vi "HFRR ADV v010new software.vi"() -> ()   [LabVIEW 2025] (continued)
              n1799 = String Subset(string=w2117, offset (0)=45, length (rest)=9 ("length (rest)")) -> (substring=w2132:string)
              n1800 = String Subset(string=w2117, offset (0)=65, length (rest)=9 ("length (rest)")) -> (substring=w2138:string)
              n1801 = Fract/Exp String To Number(string=w2124) -> (number=w2121:dbl)  [unwired: 3 in, 1 out]
              n1802 = Fract/Exp String To Number(string=w2118) -> (number=w2116:dbl)  [unwired: 3 in, 1 out]
              n1803 = Fract/Exp String To Number(string=w2126) -> (number=w2125:dbl)  [unwired: 3 in, 1 out]
              n1804 = Fract/Exp String To Number(string=w2132) -> (number=w2129:dbl)  [unwired: 3 in, 1 out]
              n1805 = Fract/Exp String To Number(string=w2138) -> (number=w2135:dbl)  [unwired: 3 in, 1 out]
              n1806 = Add(x=w2135, y=0.0) -> (x+y=w2133:dbl)
            }
            n1807 = for {
              N: w1987 -> [_]
              tunnel: w1998 -> [w2078]
              tunnel: w1997 -> [w2077]
              tunnel: [w2067] -> w1956 mode=indexing
              tunnel: [w2065] -> w1954 mode=indexing
              tunnel: [w2066] -> w1950 mode=indexing
              tunnel: w1985 -> [_]
              tunnel: [w2059] -> w1952 mode=indexing
              tunnel: [w2055] -> w1934 mode=indexing
              tunnel: [w2051] -> w1910 mode=indexing
              tunnel: [w2048] -> w1891 mode=indexing
              tunnel: [w2044] -> w1850 mode=indexing
              (unwired) 9 ("length (rest)")
              (unwired) 9 ("length (rest)")
              (unwired) TRUE ("line mode (F)")
              n1808 = Read from Text File "Read File"(file (use dialog)=w2077, error in=w2078) -> (text=w2045:string)  [unwired: 2 in, 3 out]
              n1809 = local write "String 8"(w2045) -> ()
              n1810 = String Subset(string=w2045, offset (0)=85) -> (substring=w2047:string)  [unwired: 1 in]
              n1811 = String Subset(string=w2045, offset (0)=35, length (rest)=9 ("length (rest)")) -> (substring=w2068:string)
              n1812 = String Subset(string=w2045, offset (0)=55, length (rest)=9 ("length (rest)")) -> (substring=w2053:string)
              n1813 = String Subset(string=w2045, offset (0)=25) -> (substring=w2049:string)  [unwired: 1 in]
              n1814 = String Subset(string=w2045, offset (0)=15, length (rest)=9 ("length (rest)")) -> (substring=w2074:string)
              n1815 = String Subset(string=w2045, offset (0)=0, length (rest)=14 ("length (rest)")) -> (substring=w2071:string)
              n1816 = String Subset(string=w2045, offset (0)=45, length (rest)=9 ("length (rest)")) -> (substring=w2058:string)
              n1817 = String Subset(string=w2045, offset (0)=65, length (rest)=9 ("length (rest)")) -> (substring=w2064:string)
              n1818 = Fract/Exp String To Number(string=w2047) -> (number=w2044:dbl)  [unwired: 3 in, 1 out]
              n1819 = Fract/Exp String To Number(string=w2068) -> (number=w2066:dbl)  [unwired: 3 in, 1 out]
              n1820 = Fract/Exp String To Number(string=w2053) -> (number=w2051:dbl)  [unwired: 3 in, 1 out]
              n1821 = Fract/Exp String To Number(string=w2049) -> (number=w2048:dbl)  [unwired: 3 in, 1 out]
              n1822 = Fract/Exp String To Number(string=w2074) -> (number=w2065:dbl)  [unwired: 3 in, 1 out]
              n1823 = Fract/Exp String To Number(string=w2071) -> (number=w2067:dbl)  [unwired: 3 in, 1 out]
              n1824 = Fract/Exp String To Number(string=w2058) -> (number=w2055:dbl)  [unwired: 3 in, 1 out]
              n1825 = Fract/Exp String To Number(string=w2064) -> (number=w2061:dbl)  [unwired: 3 in, 1 out]
              n1826 = Add(x=w2061, y=0.0) -> (x+y=w2059:dbl)
            }
            n1827 = String To Path(string=w1904) -> (path=w2002:path)
            n1828 = String To Path(string=w1902) -> (path=w1996:path)
            n1829 = local read "Numeric 11"() -> (w1986:i32)
            n1830 = local read "Numeric 13"() -> (w1988:i32)
            n1831 = Open/Create/Replace File "Open File"(file path (use dialog)=w2002) -> (refnum out=w2000:refnum<file>, error out=w1999:errorcluster)  [unwired: 5 in, 1 out]
            n1832 = Open/Create/Replace File "Open File"(file path (use dialog)=w1996) -> (refnum out=w1995:refnum<file>, error out=w1994:errorcluster)  [unwired: 5 in, 1 out]
            n1833 = for {
              N: w1986 -> [_]
              tunnel: w2000 -> [w2115]
              tunnel: w1999 -> [w2114]
              tunnel: [w2104] -> w1966 mode=indexing
              tunnel: [w2102] -> w1964 mode=indexing
              tunnel: [w2103] -> w1959 mode=indexing
              tunnel: w1985 -> [_]
              tunnel: [w2096] -> w1961 mode=indexing
              tunnel: [w2092] -> w1937 mode=indexing
              tunnel: [w2088] -> w1912 mode=indexing
              tunnel: [w2084] -> w1893 mode=indexing
              tunnel: [w2079] -> w1851 mode=indexing
              (unwired) TRUE ("line mode (F)")
              n1834 = Read from Text File "Read File"(file (use dialog)=w2115, error in=w2114) -> (text=w2080:string)  [unwired: 2 in, 3 out]
              n1835 = local write "String 7"(w2080) -> ()
              n1836 = String Subset(string=w2080, offset (0)=85, length (rest)=9 ("length (rest)")) -> (substring=w2083:string)
              n1837 = String Subset(string=w2080, offset (0)=35, length (rest)=9 ("length (rest)")) -> (substring=w2105:string)
              n1838 = String Subset(string=w2080, offset (0)=55, length (rest)=9 ("length (rest)")) -> (substring=w2091:string)
              n1839 = String Subset(string=w2080, offset (0)=25, length (rest)=9 ("length (rest)")) -> (substring=w2085:string)
              n1840 = String Subset(string=w2080, offset (0)=45, length (rest)=9 ("length (rest)")) -> (substring=w2093:string)
              n1841 = String Subset(string=w2080, offset (0)=0, length (rest)=14 ("length (rest)")) -> (substring=w2108:string)
              n1842 = String Subset(string=w2080, offset (0)=15, length (rest)=9 ("length (rest)")) -> (substring=w2111:string)
              n1843 = String Subset(string=w2080, offset (0)=65, length (rest)=9 ("length (rest)")) -> (substring=w2097:string)
              n1844 = Fract/Exp String To Number(string=w2083) -> (number=w2079:dbl)  [unwired: 3 in, 1 out]
              n1845 = Fract/Exp String To Number(string=w2105) -> (number=w2103:dbl)  [unwired: 3 in, 1 out]
              n1846 = Fract/Exp String To Number(string=w2091) -> (number=w2088:dbl)  [unwired: 3 in, 1 out]
              n1847 = Fract/Exp String To Number(string=w2085) -> (number=w2084:dbl)  [unwired: 3 in, 1 out]
              n1848 = Fract/Exp String To Number(string=w2093) -> (number=w2092:dbl)  [unwired: 3 in, 1 out]
              n1849 = Fract/Exp String To Number(string=w2108) -> (number=w2104:dbl)  [unwired: 3 in, 1 out]
              n1850 = Fract/Exp String To Number(string=w2111) -> (number=w2102:dbl)  [unwired: 3 in, 1 out]
              n1851 = Fract/Exp String To Number(string=w2097) -> (number=w2100:dbl)  [unwired: 3 in, 1 out]
              n1852 = Add(x=w2100, y=0.0) -> (x+y=w2096:dbl)
            }
            n1853 = for {
              N: w1988 -> [_]
              tunnel: w1995 -> [w2043]
              tunnel: w1994 -> [w2042]
              tunnel: [w2032] -> w1948 mode=indexing
              tunnel: [w2031] -> w1941 mode=indexing
              tunnel: w1985 -> [_]
              tunnel: [w2020] -> w1946 mode=indexing
              tunnel: [w2025] -> w1943 mode=indexing
              tunnel: [w2021] -> w1933 mode=indexing
              tunnel: [w2016] -> w1908 mode=indexing
              tunnel: [w2012] -> w1889 mode=indexing
              tunnel: [w2007] -> w1849 mode=indexing
              (unwired) 1.0 ("x")
              (unwired) TRUE ("line mode (F)")
              n1854 = Read from Text File "Read File"(file (use dialog)=w2043, error in=w2042) -> (text=w2008:string)  [unwired: 2 in, 3 out]
              n1855 = local write "String 12"(w2008) -> ()
              n1856 = String Subset(string=w2008, offset (0)=85, length (rest)=9 ("length (rest)")) -> (substring=w2010:string)
              n1857 = String Subset(string=w2008, offset (0)=35, length (rest)=9 ("length (rest)")) -> (substring=w2033:string)
              n1858 = String Subset(string=w2008, offset (0)=55, length (rest)=9 ("length (rest)")) -> (substring=w2018:string)
              n1859 = String Subset(string=w2008, offset (0)=25, length (rest)=9 ("length (rest)")) -> (substring=w2014:string)
              n1860 = String Subset(string=w2008, offset (0)=45, length (rest)=9 ("length (rest)")) -> (substring=w2023:string)
              n1861 = String Subset(string=w2008, offset (0)=15, length (rest)=9 ("length (rest)")) -> (substring=w2039:string)
              n1862 = String Subset(string=w2008, offset (0)=0, length (rest)=14 ("length (rest)")) -> (substring=w2036:string)
              n1863 = String Subset(string=w2008, offset (0)=65, length (rest)=9 ("length (rest)")) -> (substring=w2026:string)
              n1864 = Fract/Exp String To Number(string=w2010) -> (number=w2007:dbl)  [unwired: 3 in, 1 out]
              n1865 = Fract/Exp String To Number(string=w2033) -> (number=w2031:dbl)  [unwired: 3 in, 1 out]
              n1866 = Fract/Exp String To Number(string=w2018) -> (number=w2016:dbl)  [unwired: 3 in, 1 out]
              n1867 = Fract/Exp String To Number(string=w2014) -> (number=w2012:dbl)  [unwired: 3 in, 1 out]
              n1868 = Fract/Exp String To Number(string=w2023) -> (number=w2021:dbl)  [unwired: 3 in, 1 out]
              n1869 = Fract/Exp String To Number(string=w2039) -> (number=w2020:dbl)  [unwired: 3 in, 1 out]
              n1870 = Fract/Exp String To Number(string=w2036) -> (number=w2032:dbl)  [unwired: 3 in, 1 out]
              n1871 = Fract/Exp String To Number(string=w2026) -> (number=w2029:dbl)  [unwired: 3 in, 1 out]
              n1872 = Add(x=w2029, y=0.0) -> (x+y=w2025:dbl)
            }
            n1873 = Delete From Array(array=w1891, index=0) -> (array with subset deleted=w1864:dbl[])  [unwired: 1 in, 1 out]
            n1874 = Delete From Array(array=w1954, index=0) -> (array with subset deleted=w1927:dbl[])  [unwired: 1 in, 1 out]
            n1875 = Delete From Array(array=w1934, index=0) -> (array with subset deleted=w1922:dbl[])  [unwired: 1 in, 1 out]
            n1876 = Delete From Array(array=w1952, index=0) -> (array with subset deleted=w1953:dbl[])  [unwired: 1 in, 1 out]
            n1877 = call-poly <vilib>:"Mean.vi"("X"=w1864) -> ("mean"=→"КОФ2 4":dbl)  [unwired: 1 out]
            n1878 = call-poly <vilib>:"Mean.vi"("X"=w1927) -> ("mean"=→"КОФ3":dbl)  [unwired: 1 out]
            n1879 = call-poly <vilib>:"Mean.vi"("X"=w1922) -> ("mean"=→"CP3":dbl)  [unwired: 1 out]
            n1880 = Delete From Array(array=w1916, index=0) -> (array with subset deleted=w1843:dbl[])  [unwired: 1 in, 1 out]
            n1881 = Delete From Array(array=w1855, index=0) -> (array with subset deleted=w1842:dbl[])  [unwired: 1 in, 1 out]
            n1882 = Delete From Array(array=w1895, index=0) -> (array with subset deleted=w1866:dbl[])  [unwired: 1 in, 1 out]
            n1883 = Delete From Array(array=w1973, index=0) -> (array with subset deleted=w1928:dbl[])  [unwired: 1 in, 1 out]
            n1884 = Delete From Array(array=w1939, index=0) -> (array with subset deleted=w1924:dbl[])  [unwired: 1 in, 1 out]
            "array w/ subset deleted" <- w1924
            n1885 = Delete From Array(array=w1970, index=0) -> (array with subset deleted=w1971:dbl[])  [unwired: 1 in, 1 out]
            n1886 = call-poly <vilib>:"Mean.vi"("X"=w1866) -> ("mean"=→"КОФ2 2":dbl)  [unwired: 1 out]
            n1887 = call-poly <vilib>:"Mean.vi"("X"=w1928) -> ("mean"=→"КОФ1":dbl)  [unwired: 1 out]
            n1888 = Bundle "Bundle"(w1843, w1842) -> (w1848:cluster{dbl[], dbl[]})  [unwired: 1 in]
            n1889 = Bundle "Bundle"(w1843, w1971) -> (w1835:cluster{dbl[], dbl[]})  [unwired: 1 in]
            n1890 = Delete From Array(array=w1850, index=0) -> (array with subset deleted=w1838:dbl[])  [unwired: 1 in, 1 out]
            n1891 = Delete From Array(array=w1851, index=0) -> (array with subset deleted=w1840:dbl[])  [unwired: 1 in, 1 out]
            n1892 = Delete From Array(array=w1961, index=0) -> (array with subset deleted=w1962:dbl[])  [unwired: 1 in, 1 out]
            n1893 = Delete From Array(array=w1849, index=0) -> (array with subset deleted=w1836:dbl[])  [unwired: 1 in, 1 out]
            n1894 = Delete From Array(array=w1943, index=0) -> (array with subset deleted=w1944:dbl[])  [unwired: 1 in, 1 out]
            n1895 = Delete From Array(array=w1968, index=0) -> (array with subset deleted=w1874:dbl[])  [unwired: 1 in, 1 out]
            n1896 = Delete From Array(array=w1914, index=0) -> (array with subset deleted=w1870:dbl[])  [unwired: 1 in, 1 out]
            n1897 = Delete From Array(array=w1950, index=0) -> (array with subset deleted=w1872:dbl[])  [unwired: 1 in, 1 out]
            n1898 = Delete From Array(array=w1910, index=0) -> (array with subset deleted=w1868:dbl[])  [unwired: 1 in, 1 out]
            n1899 = Delete From Array(array=w1959, index=0) -> (array with subset deleted=w1873:dbl[])  [unwired: 1 in, 1 out]
            n1900 = Delete From Array(array=w1912, index=0) -> (array with subset deleted=w1869:dbl[])  [unwired: 1 in, 1 out]
            n1901 = Delete From Array(array=w1893, index=0) -> (array with subset deleted=w1865:dbl[])  [unwired: 1 in, 1 out]
            n1902 = Delete From Array(array=w1937, index=0) -> (array with subset deleted=w1923:dbl[])  [unwired: 1 in, 1 out]
            n1903 = Delete From Array(array=w1964, index=0) -> (array with subset deleted=w1925:dbl[])  [unwired: 1 in, 1 out]
            n1904 = Delete From Array(array=w1941, index=0) -> (array with subset deleted=w1871:dbl[])  [unwired: 1 in, 1 out]
            n1905 = Delete From Array(array=w1908, index=0) -> (array with subset deleted=w1867:dbl[])  [unwired: 1 in, 1 out]
            n1906 = Delete From Array(array=w1889, index=0) -> (array with subset deleted=w1863:dbl[])  [unwired: 1 in, 1 out]
            n1907 = Delete From Array(array=w1933, index=0) -> (array with subset deleted=w1921:dbl[])  [unwired: 1 in, 1 out]
            n1908 = Delete From Array(array=w1946, index=0) -> (array with subset deleted=w1926:dbl[])  [unwired: 1 in, 1 out]
            n1909 = Delete From Array(array=w1956, index=0) -> (array with subset deleted=w1839:dbl[])  [unwired: 1 in, 1 out]
            n1910 = Delete From Array(array=w1966, index=0) -> (array with subset deleted=w1841:dbl[])  [unwired: 1 in, 1 out]
            n1911 = Delete From Array(array=w1948, index=0) -> (array with subset deleted=w1837:dbl[])  [unwired: 1 in, 1 out]
            n1912 = Bundle "Bundle"(w1843, w1874) -> (w1861:cluster{dbl[], dbl[]})  [unwired: 1 in]
            n1913 = Bundle "Bundle"(w1843, w1928) -> (w1862:cluster{dbl[], dbl[]})  [unwired: 1 in]
            n1914 = Bundle "Bundle"(w1874, w1870) -> (w1876:cluster{dbl[], dbl[]})  [unwired: 1 in]
            n1915 = Bundle "Bundle"(w1839, w1838) -> (w1846:cluster{dbl[], dbl[]})  [unwired: 1 in]
            n1916 = Bundle "Bundle"(w1872, w1868) -> (w1878:cluster{dbl[], dbl[]})  [unwired: 1 in]
            n1917 = Bundle "Bundle"(w1839, w1872) -> (w1982:cluster{dbl[], dbl[]})  [unwired: 1 in]
            n1918 = Bundle "Bundle"(w1839, w1868) -> (w1906:cluster{dbl[], dbl[]})  [unwired: 1 in]
            n1919 = Bundle "Bundle"(w1839, w1927) -> (w1992:cluster{dbl[], dbl[]})  [unwired: 1 in]
            n1920 = Bundle "Bundle"(w1839, w1922) -> (w1930:cluster{dbl[], dbl[]})  [unwired: 1 in]
            n1921 = Bundle "Bundle"(w1839, w1953) -> (w1977:cluster{dbl[], dbl[]})  [unwired: 1 in]
            n1922 = Bundle "Bundle"(w1873, w1869) -> (w1877:cluster{dbl[], dbl[]})  [unwired: 1 in]
            n1923 = Bundle "Bundle"(w1841, w1840) -> (w1847:cluster{dbl[], dbl[]})  [unwired: 1 in]
            n1924 = Bundle "Bundle"(w1841, w1873) -> (w1984:cluster{dbl[], dbl[]})  [unwired: 1 in]
            n1925 = Bundle "Bundle"(w1841, w1869) -> (w1907:cluster{dbl[], dbl[]})  [unwired: 1 in]
            n1926 = Bundle "Bundle"(w1841, w1923) -> (w1931:cluster{dbl[], dbl[]})  [unwired: 1 in]
            n1927 = Bundle "Bundle"(w1841, w1925) -> (w1993:cluster{dbl[], dbl[]})  [unwired: 1 in]
            n1928 = Bundle "Bundle"(w1841, w1962) -> (w1975:cluster{dbl[], dbl[]})  [unwired: 1 in]
            n1929 = Bundle "Bundle"(w1871, w1867) -> (w1879:cluster{dbl[], dbl[]})  [unwired: 1 in]
            n1930 = Bundle "Bundle"(w1837, w1836) -> (w1845:cluster{dbl[], dbl[]})  [unwired: 1 in]
            n1931 = Bundle "Bundle"(w1837, w1871) -> (w1983:cluster{dbl[], dbl[]})  [unwired: 1 in]
            n1932 = Bundle "Bundle"(w1837, w1867) -> (w1905:cluster{dbl[], dbl[]})  [unwired: 1 in]
            n1933 = Bundle "Bundle"(w1837, w1921) -> (w1929:cluster{dbl[], dbl[]})  [unwired: 1 in]
            n1934 = Bundle "Bundle"(w1837, w1926) -> (w1991:cluster{dbl[], dbl[]})  [unwired: 1 in]
            n1935 = Bundle "Bundle"(w1837, w1944) -> (w1976:cluster{dbl[], dbl[]})  [unwired: 1 in]
            n1936 = call-poly <vilib>:"Mean.vi"("X"=w1924) -> ("mean"=→"CP1":dbl)  [unwired: 1 out]
            n1937 = call-poly <vilib>:"Mean.vi"("X"=w1865) -> ("mean"=→"КОФ2 3":dbl)  [unwired: 1 out]
            n1938 = call-poly <vilib>:"Mean.vi"("X"=w1923) -> ("mean"=→"CP2":dbl)  [unwired: 1 out]
            n1939 = call-poly <vilib>:"Mean.vi"("X"=w1925) -> ("mean"=→"КОФ2":dbl)  [unwired: 1 out]
            n1940 = call-poly <vilib>:"Mean.vi"("X"=w1863) -> ("mean"=→"КОФ2 5":dbl)  [unwired: 1 out]
            n1941 = call-poly <vilib>:"Mean.vi"("X"=w1921) -> ("mean"=→"CP4":dbl)  [unwired: 1 out]
            n1942 = call-poly <vilib>:"Mean.vi"("X"=w1926) -> ("mean"=→"КОФ4":dbl)  [unwired: 1 out]
            n1943 = Bundle "Bundle"(w1843, w1870) -> (w1834:cluster{dbl[], dbl[]})  [unwired: 1 in]
            n1944 = Bundle "Bundle"(w1843, w1924) -> (w1857:cluster{dbl[], dbl[]})  [unwired: 1 in]
            n1945 = Build Array "Build Array"(w1834, w1857) -> (w1860:cluster{dbl[], dbl[]}[])
            "XY Graph 17" <- w1860
            n1946 = Build Array "Build Array"(w1848, w1847, w1846, w1845) -> (→"Frequency ( Hz )":cluster{dbl[], dbl[]}[])
            n1947 = Build Array "Build Array"(w1876, w1877, w1878, w1879) -> (→"Air Temp ( °C ) vs Humidity ( % RH )":cluster{dbl[], dbl[]}[])
            n1948 = Build Array "Build Array"(w1861, w1984, w1982, w1983) -> (→"Air Temperature  ( °C )":cluster{dbl[], dbl[]}[])
            n1949 = Build Array "Build Array"(w1834, w1907, w1906, w1905) -> (→"Humidity ( %RH )":cluster{dbl[], dbl[]}[])
            n1950 = Build Array "Build Array"(w1862, w1993, w1992, w1991) -> (→"Coefficient Of Friction":cluster{dbl[], dbl[]}[])
            n1951 = Build Array "Build Array"(w1857, w1931, w1930, w1929) -> (→"Sample Temperature ( °C )":cluster{dbl[], dbl[]}[])
            n1952 = Build Array "Build Array"(w1835, w1975, w1977, w1976) -> (→"XY Graph 13":cluster{dbl[], dbl[]}[])
            n1953 = Bundle "Bundle"(w1843, w1866) -> (w1888:cluster{dbl[], dbl[]})  [unwired: 1 in]
            n1954 = Bundle "Bundle"(w1839, w1864) -> (w1886:cluster{dbl[], dbl[]})  [unwired: 1 in]
            n1955 = Bundle "Bundle"(w1841, w1865) -> (w1887:cluster{dbl[], dbl[]})  [unwired: 1 in]
            n1956 = Bundle "Bundle"(w1837, w1863) -> (w1885:cluster{dbl[], dbl[]})  [unwired: 1 in]
            n1957 = Build Array "Build Array"(w1888, w1887, w1886, w1885) -> (→"Stroke ( mm )":cluster{dbl[], dbl[]}[])
            n1958 = local write "XY Graph 16"(w1860) -> ()
          }
          frame #2 {
          }
          frame #3 {
            n1959 = local write "Numeric 8"(0 ("Numeric 8")) -> ()
            n1960 = local write "Numeric 11"(0 ("Numeric 11")) -> ()
            n1961 = local write "Numeric 12"(0 ("Numeric 12")) -> ()
            n1962 = local write "Numeric 13"(0 ("Numeric 13")) -> ()
            n1963 = property on="OPEN" class="Bool (strict)"("Visible"=TRUE) -> ()  [unwired: 2 in, 2 out]
            n1964 = local read "String Control 2"() -> (w2160:string)
            n1965 = local read "String Control 4"() -> (w2159:string)
            n1966 = local read "String Control 6"() -> (w2158:string)
            n1967 = local read "String Control 8"() -> (w2157:string)
            n1968 = Match Pattern(string=w2160, regular expression="Samples / cycle :- ") -> (after substring=w2174:string)  [unwired: 1 in, 3 out]
            n1969 = Match Pattern(string=w2160, regular expression="Frequency :- ") -> (after substring=w2193:string)  [unwired: 1 in, 3 out]
            n1970 = Match Pattern(string=w2159, regular expression="Samples / cycle :- ") -> (after substring=w2170:string)  [unwired: 1 in, 3 out]
            n1971 = Match Pattern(string=w2159, regular expression="Frequency :- ") -> (after substring=w2188:string)  [unwired: 1 in, 3 out]
            n1972 = Match Pattern(string=w2158, regular expression="Samples / cycle :- ") -> (after substring=w2166:string)  [unwired: 1 in, 3 out]
            n1973 = Match Pattern(string=w2158, regular expression="Frequency :- ") -> (after substring=w2183:string)  [unwired: 1 in, 3 out]
            n1974 = Match Pattern(string=w2157, regular expression="Samples / cycle :- ") -> (after substring=w2162:string)  [unwired: 1 in, 3 out]
            n1975 = Match Pattern(string=w2157, regular expression="Frequency :- ") -> (after substring=w2178:string)  [unwired: 1 in, 3 out]
            n1976 = String Subset(string=w2174, length (rest)=6 ("length (rest)")) -> (substring=w2176:string)  [unwired: 1 in]
            n1977 = String Subset(string=w2193, length (rest)=9 ("length (rest)")) -> (substring=w2195:string)  [unwired: 1 in]
            n1978 = String Subset(string=w2170, length (rest)=6 ("length (rest)")) -> (substring=w2172:string)  [unwired: 1 in]
            n1979 = String Subset(string=w2188, length (rest)=9 ("length (rest)")) -> (substring=w2190:string)  [unwired: 1 in]
            n1980 = String Subset(string=w2166, length (rest)=6 ("length (rest)")) -> (substring=w2168:string)  [unwired: 1 in]
            n1981 = String Subset(string=w2183, length (rest)=9 ("length (rest)")) -> (substring=w2185:string)  [unwired: 1 in]
            n1982 = String Subset(string=w2162, length (rest)=6 ("length (rest)")) -> (substring=w2164:string)  [unwired: 1 in]
            n1983 = String Subset(string=w2178, length (rest)=9 ("length (rest)")) -> (substring=w2180:string)  [unwired: 1 in]
            n1984 = Fract/Exp String To Number(string=w2176) -> (number=w2156:dbl)  [unwired: 3 in, 1 out]
            n1985 = Fract/Exp String To Number(string=w2195) -> (number=w2196:dbl)  [unwired: 3 in, 1 out]
            n1986 = Fract/Exp String To Number(string=w2172) -> (number=w2155:dbl)  [unwired: 3 in, 1 out]
            n1987 = Fract/Exp String To Number(string=w2190) -> (number=w2191:dbl)  [unwired: 3 in, 1 out]
            n1988 = Fract/Exp String To Number(string=w2168) -> (number=w2154:dbl)  [unwired: 3 in, 1 out]
            n1989 = Fract/Exp String To Number(string=w2185) -> (number=w2186:dbl)  [unwired: 3 in, 1 out]
            n1990 = Fract/Exp String To Number(string=w2164) -> (number=w2153:dbl)  [unwired: 3 in, 1 out]
            n1991 = Fract/Exp String To Number(string=w2180) -> (number=w2181:dbl)  [unwired: 3 in, 1 out]
            n1992 = local write "sample1"(w2156) -> ()
            n1993 = local write "freq1"(w2196) -> ()
            n1994 = local write "sample2"(w2155) -> ()
            n1995 = local write "freq2"(w2191) -> ()
            n1996 = local write "sample3"(w2154) -> ()
            n1997 = local write "freq3"(w2186) -> ()
            n1998 = local write "sample4"(w2153) -> ()
            n1999 = local write "freq 4"(w2181) -> ()
          }
        }
      }
    }
    n2000 = case shown="True" w1645 {
      selector: w1645 -> [_ w1773]
      frame False {
      }
      frame True {
        n2001 = Not(x=w1773) -> (.not. x?=w1769:bool)
        n2002 = local write "service 3"(w1769) -> ()
        n2003 = local write "OPEN 6"(w1769) -> ()
        n2004 = call <vilib>:"System Exec.vi"("wait until completion? (T)"=TRUE, "command line"="C:\\LAB-IQ\\Scar View.exe") -> ("error out"=→"error out 5":errorcluster)  [unwired: 6 in, 3 out]
      }
    }
    n2005 = case shown="\"Acquire\", Default" w1656 {
      frame "Acquire", Default {
        w2669 = 0.2 ("y")
        w2674 = 1.0 ("y")
        w2675 = 0.8 ("y")
        # "Elapsed time\ncof\nstroke\nAir temp\nTemp\nHumidity"
        n2006 = disable-structure shown="Disabled" {
          frame Disabled {
            n2007 = local read "Flag"() -> (w2692:dbl)
            n2008 = local read "RUN"() -> (w2689:bool)
            n2009 = Not(x=w2689) -> (.not. x?=w2688:bool)
            n2010 = Equal?(x=w2692, y=10.0) -> (x = y?=w2690:bool)
            n2011 = And(x=w2690, y=w2688) -> (x .and. y?=w2687:bool)
            n2012 = case shown="True" w2687 {
              frame False {
              }
              frame True {
                w2693 = FALSE ("Heater Button")
                n2013 = local write "Humidity"(w2693) -> ()
                n2014 = local write "Heater Button"(w2693) -> ()
              }
            }
          }
          frame Enabled {
          }
        }
        n2015 = disable-structure shown="Disabled" {
          frame Disabled {
            n2016 = case shown="True" {
              selector: _ -> [_ _]
              frame False {
              }
              frame True {
                w2784 = TRUE ("Heater")
                n2017 = local write "Humidity"(w2784) -> ()
                n2018 = local write "Heater Button"(w2784) -> ()
                n2019 = local read "TEST STANDARD"() -> (w2787:T3)
                n2020 = local read "TEST STANDARD"() -> (w2782:T3)
                n2021 = Equal?(x=w2787, y=enum16{"ASTM D6079", "ISO 12156", "Custom"}."ISO 12156" ("Test Standard")) -> (x = y?=w2785:bool)
                n2022 = Equal?(x=w2782, y=enum16{"ASTM D6079", "ISO 12156", "Custom"}."ASTM D6079" ("Test Standard")) -> (x = y?=w2781:bool)
                n2023 = case shown="True" w2785 {
                  frame False {
                  }
                  frame True {
                    n2024 = local write "Heater"(TRUE ("Heater")) -> ()
                    n2025 = local write "airtempflg"(FALSE ("airtempflg")) -> ()
                  }
                }
                n2026 = case shown="True" w2781 {
                  frame False {
                  }
                  frame True {
                    n2027 = local write "Heater"(FALSE ("Heater")) -> ()
                    n2028 = local write "airtempflg"(TRUE ("airtempflg")) -> ()
                  }
                }
              }
            }
          }
          frame Enabled {
          }
        }
        n2029 = stacked-sequence {
          frame #0 {
            n2030 = case shown="True" "RST FF" {
              frame False {
              }
              frame True {
                w2850 = 0.0 ("X Scale.Range:Maximum")
                n2031 = property on="Frictional Force ( N )" class="WFChart (strict)"("XScale.Maximum"=600.0 ("X Scale.Range:Maximum"), "XScale.Minimum"=w2850, "YScale.Maximum"=10.0 ("Y Scale.Range:Maximum"), "YScale.Minimum"=w2850) -> ()  [unwired: 2 in, 2 out]
              }
            }
          }
          frame #1 {
            n2032 = case shown="True" "RST TEMP" {
              frame False {
              }
              frame True {
                n2033 = property on="Temperature ( Deg C )" class="WFChart (strict)"("XScale.Minimum"=0.0 ("X Scale.Range:Minimum"), "XScale.Maximum"=600.0 ("X Scale.Range:Maximum"), "YScale.Minimum"=0.0 ("Y Scale.Range:Minimum"), "YScale.Maximum"=100.0 ("Y Scale.Range:Maximum")) -> ()  [unwired: 2 in, 2 out]
              }
            }
          }
          frame #2 {
            n2034 = case shown="True" "RSTCOF" {
              frame False {
              }
              frame True {
                n2035 = property on="Coefficient of Friction" class="WFChart (strict)"("XScale.Minimum"=0.0 ("X Scale.Range:Minimum"), "XScale.Maximum"=600.0 ("X Scale.Range:Maximum"), "YScale.Maximum"=1.0 ("X Scale.Range:Minimum"), "YScale.Minimum"=0.0 ("X Scale.Range:Minimum")) -> ()  [unwired: 2 in, 2 out]
              }
            }
          }
          frame #3 {
            n2036 = case shown="True" "RSTCOF 2" {
              frame False {
              }
              frame True {
                (unwired) 100.0 ("Y Scale.Range:Maximum")
                (unwired) 0.0 ("Y Scale.Range:Minimum")
                (unwired) 600.0 ("X Scale.Range:Maximum")
                (unwired) 0.0 ("X Scale.Range:Minimum")
              }
            }
          }
          frame #4 {
            n2037 = case shown="True" "RSTCOF 3" {
              frame False {
              }
              frame True {
                n2038 = property on="Electrical Contact Resistance ( % )" class="WFChart (strict)"("XScale.Minimum"=0.0 ("X Scale.Range:Minimum"), "XScale.Maximum"=600.0 ("X Scale.Range:Maximum"), "YScale.Minimum"=0.0 ("Y Scale.Range:Minimum"), "YScale.Maximum"=100.0 ("Y Scale.Range:Maximum")) -> ()  [unwired: 2 in, 2 out]
              }
            }
          }
        }
        n2039 = disable-structure shown="Disabled" {
          frame Disabled {
            n2040 = case shown="True" {
              selector: _ -> [_ _]
              frame False {
              }
              frame True {
                n2041 = local read "zflag 2"() -> (w2751:dbl)
                n2042 = local read "yflag"() -> (w2753:dbl)
                n2043 = Equal?(x=w2753, y=2.0 ("tflag")) -> (x = y?=w2755:bool)
                n2044 = Equal?(x=w2751, y=3.0 ("tflag")) -> (x = y?=w2754:bool)
                n2045 = And(x=w2755, y=w2754) -> (x .and. y?=w2749:bool)
                n2046 = case shown="True" w2749 {
                  frame False {
                  }
                  frame True {
                    w2780 = 0.0 ("zflag")
                    n2047 = local write "zflag"(w2780) -> ()
                    n2048 = local write "zflag 2"(w2780) -> ()
                    n2049 = Delete(path (use dialog)=path "C:/LAB-IQ-NXT/WO 2449 TT.sig" ("file path (dialog if empty)")) -> (deleted path=w2779:path)  [unwired: 4 in, 2 out]
                    n2050 = Delete(path (use dialog)=path "C:/LAB-IQ-NXT/WO 2449 TRH.sig" ("file path (dialog if empty)")) -> (deleted path=w2774:path)  [unwired: 4 in, 2 out]
                    n2051 = local read "SEN.RUN HRS"() -> (w2766:dbl)
                    n2052 = local read "SENSOR TIME"() -> (w2764:dbl)
                    n2053 = call <vilib>:"compatOverwrite.vi"("overwrite (F)"=TRUE) -> ("overwrite?"=w2756:T29)
                    n2054 = call <vilib>:"compatOverwrite.vi"("overwrite (F)"=TRUE) -> ("overwrite?"=w2760:T29)
                    n2055 = local read "Total No. of Tests"() -> (w2767:dbl)
                    n2056 = Add(x=w2764, y=w2766) -> (x+y=w2765:dbl)
                    "SEN.RUN HRS" <- w2765
                    n2057 = Open/Create/Replace File(file path (use dialog)=w2779, operation (0:open)=w2756) -> (refnum out=w2757:refnum<file>, error out=w2758:errorcluster)  [unwired: 4 in, 1 out]
                    n2058 = Open/Create/Replace File(file path (use dialog)=w2774, operation (0:open)=w2760) -> (refnum out=w2761:refnum<file>, error out=w2762:errorcluster)  [unwired: 4 in, 1 out]
                    n2059 = Deny Access(4:w2758, 6:T27."deny none" ("deny mode (2)"), 7:w2757) -> (3:w2778:refnum<file>)  [unwired: 1 out]
                    n2060 = Deny Access(4:w2762, 6:T27."deny none" ("deny mode (2)"), 7:w2761) -> (3:w2770:refnum<file>)  [unwired: 1 out]
                    n2061 = Number To Decimal String(number=w2767) -> (decimal integer string=w2775:string)  [unwired: 1 in]
                    n2062 = Number To Decimal String(number=w2765) -> (decimal integer string=w2771:string)  [unwired: 1 in]
                    n2063 = Write to Binary File(file (use dialog)=w2778, data=w2775, 5:FALSE ("prepend array or string size? (T)")) -> ()  [unwired: 3 in, 3 out]
                    n2064 = Write to Binary File(file (use dialog)=w2770, data=w2771, 5:FALSE ("prepend array or string size? (T)")) -> ()  [unwired: 3 in, 3 out]
                  }
                }
              }
            }
          }
          frame Enabled {
          }
        }
        n2065 = local read "RUN"() -> (w2678:bool)
        n2066 = local read "run replace"() -> (w2682:bool)
        n2067 = local read "run replace"() -> (w2681:bool)
        n2068 = case shown="True" w2678 {
          frame False {
            n2069 = local write "run replace"(FALSE ("run replace")) -> ()
          }
          frame True {
            "run replace" <- TRUE ("run replace")
          }
        }
        n2070 = local read "RUN"() -> (w2686:bool)
        n2071 = local read "Set Temp"() -> (w2648:dbl)
        n2072 = local read "SetTemp"() -> (w2650:dbl)
        n2073 = case shown="False" w2686 {
          tunnel: [FALSE ("TEST RUNNING") TRUE ("TEST RUNNING")] -> w2685
          frame False {
            w2869 = 0.0 ("Flag")
            n2074 = local write "Elapsed time"(0.0 ("elapsedtime")) -> ()
            n2075 = local write "Time Remaining"(w2869) -> ()
            n2076 = local write "Flag"(w2869) -> ()
            n2077 = local write "Remaining Time"(w2869) -> ()
          }
          frame True {
            n2078 = local write "Flag"(10.0 ("Flag")) -> ()
          }
        }
        n2079 = case shown="False" w2682 {
          frame False {
            n2080 = local read "zflag"() -> (→"zflag 2":dbl)
            n2081 = local write "yflag"(2.0 ("tflag")) -> ()
            n2082 = local write "FLAG 4"(0.0 ("FLAG")) -> ()
          }
          frame True {
            n2083 = local write "yflag"(1.0 ("tflag")) -> ()
            n2084 = local write "zflag"(3.0 ("zflag")) -> ()
          }
        }
        n2085 = local read "acq 2"() -> (w2680:bool)
        n2086 = local read "AIR TEMP"() -> (w2643:dbl)
        n2087 = local read "Amb temp"() -> (w2647:dbl)
        n2088 = case shown="True" "Save & Continue" {
          frame False {
          }
          frame True {
            "acq 2" <- TRUE ("acq 2")
          }
        }
        n2089 = local read "Set Rh"() -> (w2649:dbl)
        n2090 = Add(x=w2650, y=w2675) -> (x+y=w2676:dbl)
        n2091 = Subtract(x=w2650, y=w2675) -> (x-y=w2677:dbl)
        n2092 = Add(x=w2648, y=w2669) -> (x+y=w2670:dbl)
        n2093 = Subtract(x=w2648, y=w2669) -> (x-y=w2671:dbl)
        n2094 = And(x=w2680, y=w2681) -> (x .and. y?=w2679:bool)
        n2095 = Greater Or Equal?(x=w2643, y=15.0) -> (x >= y?=w2644:bool)
        "powstat" <- w2644
        n2096 = local read "Humidity ( %RH )"() -> (w2646:dbl)
        n2097 = case shown="True" "Save & Continue" {
          frame False {
          }
          frame True {
            n2098 = while {
              tunnel: "0123456789abcdefghijklmnopqrstuvwxyzABCDEFGHIJKLMNOPQRSTUVWXYZ" ("string 2") -> [w2840]
              shift-right: [w2838] -> w2833
              shift-left: "" -> [w2837]
              i -> [w2847]
              stop <- w2846 stop-if-true
              n2099 = Random Number (0-1)() -> (number: 0 to 1=w2841:dbl)
              n2100 = Multiply(x=w2841, y=62.0) -> (x*y=w2843:dbl)
              n2101 = Decrement(x="Length") -> (x-1=w2836:i16)
              n2102 = To Word Integer(number=w2843) -> (16bit integer=w2844:i16)
              n2103 = String Subset(string=w2840, offset (0)=w2844, length (rest)=1 ("length (rest)")) -> (substring=w2839:string)
              n2104 = Greater Or Equal?(x=w2847, y=w2836) -> (x >= y?=w2846:bool)
              n2105 = Concatenate Strings(w2839, w2837) -> (w2838:string)
            }
            n2106 = local write "UUID"(w2833) -> ()
          }
        }
        n2107 = In Range and Coerce(upper limit=w2676, x=w2647, lower limit=w2677) -> (In Range?=w2666:bool)  [unwired: 1 out]
        n2108 = Add(x=w2649, y=w2674) -> (x+y=w2673:dbl)
        n2109 = Subtract(x=w2649, y=w2674) -> (x-y=w2672:dbl)
        n2110 = local read "TEMP"() -> (w2645:dbl)
        n2111 = case shown="True" "Save & Continue" {
          frame False {
          }
          frame True {
            n2112 = local read "Operator ID"() -> (w3157:string)
            n2113 = local read "FILE"() -> (w3163:string)
            n2114 = String Length(string=w3163) -> (length=w3161:i32)
            n2115 = String Length(string=w3157) -> (length=w3158:i32)
            n2116 = Greater?(x=w3161, y=0) -> (0:w3160:bool)
            n2117 = Greater?(x=w3158, y=0) -> (0:w3156:bool)
            n2118 = And(x=w3160, y=w3156) -> (x .and. y?=w3155:bool)
            n2119 = case shown="True" w3155 {
              frame False {
                n2120 = stacked-sequence {
                  frame #0 {
                    n2121 = One Button Dialog(message="Please Enter a File Name and Operator ID to save data !", button name ("OK")="Ok") -> ()  [unwired: 1 out]
                  }
                  frame #1 {
                    n2122 = local write "Save & Continue"(FALSE ("OK Button")) -> ()
                  }
                }
                n2123 = local write "Save & Continue"(FALSE ("OK Button")) -> ()
              }
              frame True {
                n2124 = stacked-sequence {
                  frame #0 {
                    n2125 = local read "FILE"() -> (w3169:string)
                    n2126 = call "file check.vi"("file name in"=w3169) -> ("file name out"=w3168:string)  [unwired: 9 in, 1 out]
                    n2127 = call <vilib>:"Application Directory.vi"() -> ("Application Directory"=w3179:path)
                    n2128 = Build Path(base path=w3179, name or relative path="data") -> (appended path=w3178:path)
                    n2129 = call <vilib>:"Trim Whitespace.vi"("string"=w3168) -> ("trimmed string"=w3176:string)  [unwired: 1 in]
                    n2130 = call <vilib>:"Trim Whitespace.vi"("string"=w3168) -> ("trimmed string"=w3177:string)  [unwired: 1 in]
                    n2131 = List Folder(path=w3178) -> (folder names=w3174:string[])  [unwired: 3 in, 3 out]
                    n2132 = Match Pattern(string=w3176, regular expression="_(") -> (before substring=w3173:string)  [unwired: 1 in, 3 out]
                    n2133 = for {
                      tunnel: w3174 -> [w3188] mode=indexing
                      tunnel: w3173 -> [w3186]
                      shift-right: [w3184] -> w3171
                      shift-left: bool[] [] -> [w3185]
                      n2134 = Match Pattern(string=w3188, regular expression="_(") -> (before substring=w3187:string)  [unwired: 1 in, 3 out]
                      n2135 = Equal?(x=w3187, y=w3186) -> (x = y?=w3183:bool)
                      n2136 = case shown="True" w3183 {
                        tunnel: w3183 -> [_ w3191]
                        tunnel: w3185 -> [w3190 w3193]
                        tunnel: [w3190 w3192] -> w3184
                        frame False {
                        }
                        frame True {
                          n2137 = Insert Into Array(array=w3193, new element=w3191) -> (w3192:bool[])  [unwired: 1 in]
                        }
                      }
                    }
                    n2138 = Equal?(x=w3174, y=w3173) -> (x = y?=w3182:bool[])
                    n2139 = Or Array Elements(Boolean array=w3182) -> (logical OR=w3181:bool)
                    n2140 = Array Size(array=w3171) -> (size(s)=w3170:i32)
                    n2141 = case shown="True" w3181 {
                      tunnel: w3177 -> [_ w3201]
                      tunnel: w3170 -> [_ w3194]
                      frame False {
                      }
                      frame True {
                        n2142 = Number To Decimal String(number=w3194) -> (decimal integer string=w3197:string)  [unwired: 1 in]
                        n2143 = Search/Split String(string=w3201, search string/char (-)="_(" ("regular expression")) -> (substring before match=w3199:string)  [unwired: 1 in, 2 out]
                        n2144 = Concatenate Strings(w3199, "_(" ("regular expression"), w3197, ")" ("regular expression")) -> (w3195:string)
                        n2145 = local write "FILE"(w3195) -> ()
                      }
                    }
                  }
                  frame #1 {
                    w3203 = 0.0
                    w3216 = cluster{"y":dbl, dbl, "y":dbl}[] [] ("History Data")
                    w3217 = FALSE ("Heater Button")
                    (unwired) ")!" ("string")
                    (unwired) ")" ("string")
                    w3215 = dbl[] [] ("History Data")
                    w3221 = "\r"
                    # "C:\\WinDucom\\Data\\"
                    # "C:\\LAB-IQ-NXT\\data"
                    n2146 = local write "Humidity ( %RH )"(w3203) -> ()
                    n2147 = local write "Frequency ( Hz )"(w3203) -> ()
                    n2148 = local write "Stroke 3"(w3203) -> ()
                    n2149 = local write "speedop"(0.0 ("PIDclk 2")) -> ()
                    n2150 = local write "Set Temp 2"(65.0 ("Set Temp 2")) -> ()
                    n2151 = local write "AIR TEMP"(w3203) -> ()
                    n2152 = local write "clk"(0.0 ("clk")) -> ()
                    n2153 = local write "Stroke 4"(w3203) -> ()
                    n2154 = local write "COF 2"(w3203) -> ()
                    n2155 = local write "TEMP"(w3203) -> ()
                    n2156 = local write "ecr 3"(w3203) -> ()
                    n2157 = local write "FF 3"(w3203) -> ()
                    n2158 = local write "FF 2"(w3203) -> ()
                    n2159 = property on="Humidity ( %RH )" class="WFChart (strict)"("History Data"=w3215) -> ()  [unwired: 2 in, 2 out]
                    n2160 = property on="Coefficient of Friction" class="WFChart (strict)"("History Data"=w3215) -> ()  [unwired: 2 in, 2 out]
                    n2161 = property on="Coefficient of Friction" class="WFChart (strict)"("History Data"=w3215) -> ()  [unwired: 2 in, 2 out]
                    n2162 = property on="Frictional Force ( N )" class="WFChart (strict)"("History Data"=w3215) -> ()  [unwired: 2 in, 2 out]
                    n2163 = property on="Electrical Contact Resistance ( % )" class="WFChart (strict)"("History Data"=w3215) -> ()  [unwired: 2 in, 2 out]
                    n2164 = property on="Electrical Contact Resistance ( % )" class="WFChart (strict)"("History Data"=w3215) -> ()  [unwired: 2 in, 2 out]
                    n2165 = property on="Temperature ( Deg C )" class="WFChart (strict)"("History Data"=w3215) -> ()  [unwired: 2 in, 2 out]
                    n2166 = property on="Frictional Force ( N )" class="WFChart (strict)"("History Data"=w3215) -> ()  [unwired: 2 in, 2 out]
                    n2167 = property on="Coefficient of Friction" class="WFChart (strict)"("History Data"=w3215) -> ()  [unwired: 2 in, 2 out]
                    n2168 = property on="Frictional Force ( N )" class="WFChart (strict)"("History Data"=w3215) -> ()  [unwired: 2 in, 2 out]
                    n2169 = property on="Electrical Contact Resistance ( % )" class="WFChart (strict)"("History Data"=w3215) -> ()  [unwired: 2 in, 2 out]
                    n2170 = property on="Temperature ( Deg C )" class="WFChart (strict)"("History Data"=w3215) -> ()  [unwired: 2 in, 2 out]
                    n2171 = property on="Humidity ( %RH )" class="WFChart (strict)"("History Data"=w3215) -> ()  [unwired: 2 in, 2 out]
                    n2172 = property on="Stroke ( mm )" class="WFChart (strict)"("History Data"=w3216) -> ()  [unwired: 2 in, 2 out]
                    n2173 = property on="Stroke ( mm )" class="WFChart (strict)"("History Data"=w3216) -> ()  [unwired: 2 in, 2 out]
                    n2174 = local write "Humidity"(w3217) -> ()
                    n2175 = local write "Heater Button"(w3217) -> ()
                    n2176 = local read "FILE"() -> (w3211:string)
                    n2177 = disable-structure shown="Enabled" {
                      disable-tunnel: [w3256 _] -> w3202
                      frame Enabled {
                        n2178 = local read "NORMAL LOAD"() -> (w3256:dbl)
                      }
                      frame Disabled {
                      }
                    }
                    n2179 = call "file check.vi"("file name in"=w3211) -> ("error out"=w3214:errorcluster, "file name out"=w3208:string)  [unwired: 9 in]
                    n2180 = call "FILE PATH CREATION.vi"("error in"=w3214, "FILE NAME :"=w3208) -> ("FILE OUT"=w3207:path)  [unwired: 8 in, 1 out]
                    n2181 = Concatenate Strings(w3208, ".dgf" ("Substring")) -> (w3213:string)
                    n2182 = Concatenate Strings(w3208, ".duf" ("Substring")) -> (w3209:string)
                    n2183 = Multiply(x=w3202, y=1.0) -> (x*y=w3235:dbl)
                    n2184 = Build Path(base path=w3207, name or relative path=w3213) -> (appended path=w3206:path)
                    n2185 = Build Path(base path=w3207, name or relative path=w3209) -> (appended path=w3205:path)
                    n2186 = Number To Fractional String(number=w3235, width (-)=i16 5, precision (6)=i16 2) -> (F-format string=w3243:string)  [unwired: 1 in]
                    n2187 = local read "Fuel Discription :"() -> (w3231:string)
                    n2188 = local read "Batch Ref Num :"() -> (w3219:string)
                    n2189 = Get Date/Time String(date format (0)=enum16{"short", "long", "abbreviated"}."short") -> (date string=w3254:string, time string=w3251:string)  [unwired: 2 in]
                    n2190 = local read "Remarks :"() -> (w3230:string)
                    n2191 = Concatenate Strings("Load :- " ("Substring"), w3243, " grams ," ("Substring")) -> (w3242:string)
                    n2192 = local read "String 41"() -> (w3222:string)
                    n2193 = Concatenate Strings(w3231) -> (w3232:string)
                    n2194 = Concatenate Strings(w3219) -> (w3218:string)
                    n2195 = Concatenate Strings("tested by") -> (w3226:string)
                    n2196 = Concatenate Strings("(" ("Substring"), w3254, ")" ("Substring"), w3251) -> (w3224:string)
                    "concatenated string" <- w3224
                    n2197 = Concatenate Strings(w3230, "," ("string")) -> (w3229:string)
                    n2198 = Concatenate Strings("  TIME;      COF;       STROKE;     AIR TEMP;  TEMP;  HUMIDITY;  ECR; PID-OUT; FREQUENCY" ("Substring"), "\r") -> (w3238:string)
                    n2199 = Concatenate Strings(w3222, w3221, "Fuel Discription :-" ("Substring"), w3232, w3221, w3242, w3221, "Batch Ref Num :-" ("Substring"), w3218, w3221, " Remarks :- " ("Substring"), w3229, w3221, " Date :- " ("Substring"), w3224, w3221, "Tested By :-" ("Substring"), w3226) -> (w3236:string)
                    "REMARKS" <- w3236
                    n2200 = call <vilib>:"Write Characters To File.vi"("append to file? (new file:F)"=FALSE, "character string"=w3238, "file path (dialog if empty)"=w3206) -> ()  [unwired: 2 in, 1 out]
                    n2201 = call <vilib>:"Write Characters To File.vi"("append to file? (new file:F)"=FALSE, "character string"=w3236, "file path (dialog if empty)"=w3205) -> ()  [unwired: 2 in, 1 out]
                  }
                  frame #2 {
                    n2202 = local write "Cycles elapsed"(0 ("Cycles elapsed")) -> ()
                    n2203 = local write "cyclecount"(0 ("cyclecount")) -> ()
                    n2204 = local write "Save & Continue"(FALSE ("OK")) -> ()
                    n2205 = local write "autostrtflg"(TRUE ("autostrtflg")) -> ()
                    n2206 = local write "Save"(FALSE ("Save")) -> ()
                    n2207 = Get Date/Time In Seconds() -> (seconds since 1Jan1904=w3261:timestamp)
                    n2208 = To Double Precision Float(number=w3261) -> (double precision float=w3260:dbl)
                    n2209 = local write "acq timer"(w3260) -> ()
                    n2210 = One Button Dialog(message="Please ensure sample is mounted properly and machine is ready in all aspects for testing !", button name ("OK")="Ok") -> ()  [unwired: 1 out]
                  }
                  frame #3 {
                    n2211 = stacked-sequence {
                      frame #0 {
                        n2212 = local write "Main Dashboard Buttons"(T1."Dashboard" ("Main Dashboard Buttons")) -> ()
                        n2213 = local write "Main Tab"(T2."Acquire" ("Main Tab")) -> ()
                      }
                      frame #1 {
                        n2214 = local write "EVENT LOG"("" ("EVENT LOG")) -> ()
                      }
                      frame #2 {
                        n2215 = Wait (ms)(milliseconds to wait=u32 50) -> ()  [unwired: 1 out]
                      }
                      frame #3 {
                        n2216 = disable-structure shown="Disabled" {
                          frame Disabled {
                            n2217 = local read "EVENT LOG"() -> (w3273:string)
                            n2218 = call "Event Log.vi"("Content"="Test Details", "EVENT LOG"=w3273) -> ("EVENT LOG"=w3272:string)  [unwired: 8 in, 1 out]
                            n2219 = local write "EVENT LOG"(w3272) -> ()
                          }
                          frame Enabled {
                          }
                        }
                      }
                      frame #4 {
                        n2220 = Wait (ms)(milliseconds to wait=u32 50) -> ()  [unwired: 1 out]
                      }
                      frame #5 {
                        n2221 = local read "FILE"() -> (w3275:string)
                        n2222 = Concatenate Strings("File Name :" ("Content"), w3275) -> (w3276:string)
                        n2223 = local read "EVENT LOG"() -> (w3279:string)
                        n2224 = call "Event Log.vi"("Content"=w3276, "EVENT LOG"=w3279) -> ("EVENT LOG"=w3278:string)  [unwired: 8 in, 1 out]
                        n2225 = local write "EVENT LOG"(w3278) -> ()
                      }
                      frame #6 {
                        n2226 = Wait (ms)(milliseconds to wait=u32 50) -> ()  [unwired: 1 out]
                      }
                      frame #7 {
                        n2227 = local read "Batch Ref Num :"() -> (w3281:string)
                        n2228 = Concatenate Strings("Batch Ref No :" ("Content"), w3281) -> (w3282:string)
                        n2229 = local read "EVENT LOG"() -> (w3285:string)
                        n2230 = call "Event Log.vi"("Content"=w3282, "EVENT LOG"=w3285) -> ("EVENT LOG"=w3284:string)  [unwired: 8 in, 1 out]
                        n2231 = local write "EVENT LOG"(w3284) -> ()
                      }
                      frame #8 {
                        n2232 = Wait (ms)(milliseconds to wait=u32 50) -> ()  [unwired: 1 out]
                      }
                      frame #9 {
                        n2233 = local read "tested by"() -> (w3287:string)
                        n2234 = Concatenate Strings("Tested By :" ("Content"), w3287) -> (w3288:string)
                        n2235 = local read "EVENT LOG"() -> (w3291:string)
                        n2236 = call "Event Log.vi"("Content"=w3288, "EVENT LOG"=w3291) -> ("EVENT LOG"=w3290:string)  [unwired: 8 in, 1 out]
                        n2237 = local write "EVENT LOG"(w3290) -> ()
                      }
                      frame #10 {
                        n2238 = Wait (ms)(milliseconds to wait=u32 50) -> ()  [unwired: 1 out]
                      }
                      frame #11 {
                        n2239 = local read "TEST STANDARD"() -> (w3294:T3)
                        n2240 = case shown="\"ASTM D6079\", Default" w3294 {
                          tunnel: ["ASTM D6079" "ISO 12156" "CEC F-096-A-06" "Custom"] -> w3293
                          frame "ASTM D6079", Default {
                          }
                          frame "ISO 12156" {
                          }
                          frame "CEC F-096-A-06" {
                          }
                          frame "Custom" {
                          }
                        }
                        n2241 = Concatenate Strings("Test Standard :" ("Content"), w3293) -> (w3295:string)
                        n2242 = local read "EVENT LOG"() -> (w3298:string)
                        n2243 = call "Event Log.vi"("Content"=w3295, "EVENT LOG"=w3298) -> ("EVENT LOG"=w3297:string)  [unwired: 8 in, 1 out]
                        n2244 = local write "EVENT LOG"(w3297) -> ()
                      }
                      frame #12 {
                        n2245 = Wait (ms)(milliseconds to wait=u32 50) -> ()  [unwired: 1 out]
                      }
                      frame #13 {
                        n2246 = local read "Fuel Discription :"() -> (w3304:string)
                        n2247 = Concatenate Strings("Fuel Description :" ("Content"), w3304) -> (w3305:string)
                        n2248 = local read "EVENT LOG"() -> (w3308:string)
                        n2249 = call "Event Log.vi"("Content"=w3305, "EVENT LOG"=w3308) -> ("EVENT LOG"=w3307:string)  [unwired: 8 in, 1 out]
                        n2250 = local write "EVENT LOG"(w3307) -> ()
                      }
                      frame #14 {
                        n2251 = Wait (ms)(milliseconds to wait=u32 50) -> ()  [unwired: 1 out]
                      }
                      frame #15 {
                        n2252 = local read "Remarks :"() -> (w3310:string)
                        n2253 = Concatenate Strings("Remarks :" ("Content"), w3310) -> (w3311:string)
                        n2254 = local read "EVENT LOG"() -> (w3314:string)
                        n2255 = call "Event Log.vi"("Content"=w3311, "EVENT LOG"=w3314) -> ("EVENT LOG"=w3313:string)  [unwired: 8 in, 1 out]
                        n2256 = local write "EVENT LOG"(w3313) -> ()
                      }
                      frame #16 {
                        n2257 = Wait (ms)(milliseconds to wait=u32 50) -> ()  [unwired: 1 out]
                      }
                      frame #17 {
                        n2258 = local read "Operator ID"() -> (w3316:string)
                        n2259 = Concatenate Strings("Operator ID :" ("Content"), w3316) -> (w3318:string)
                        n2260 = local read "EVENT LOG"() -> (w3320:string)
                        n2261 = call "Event Log.vi"("Content"=w3318, "EVENT LOG"=w3320) -> ("EVENT LOG"=w3319:string)  [unwired: 8 in, 1 out]
                        n2262 = local write "EVENT LOG"(w3319) -> ()
                      }
                      frame #18 {
                        n2263 = Wait (ms)(milliseconds to wait=u32 50) -> ()  [unwired: 1 out]
                      }
                      frame #19 {
                        n2264 = disable-structure shown="Disabled" {
                          frame Disabled {
                            n2265 = local read "EVENT LOG"() -> (w3324:string)
                            n2266 = call "Event Log.vi"("Content"="Test Parameter", "EVENT LOG"=w3324) -> ("EVENT LOG"=w3323:string)  [unwired: 8 in, 1 out]
                            n2267 = local write "EVENT LOG"(w3323) -> ()
                          }
                          frame Enabled {
                          }
                        }
                      }
                      frame #20 {
                        n2268 = Wait (ms)(milliseconds to wait=u32 50) -> ()  [unwired: 1 out]
                      }
                      frame #21 {
                        n2269 = local read "Set Hz"() -> (w3328:dbl)
                        n2270 = Number To Fractional String(number=w3328, precision (6)=i16 2) -> (F-format string=w3327:string)  [unwired: 2 in]
                        n2271 = Concatenate Strings("Set Frequency [Hz] :" ("Content"), w3327) -> (w3330:string)
                        n2272 = local read "EVENT LOG"() -> (w3332:string)
